vi "Github Demo Test VI.vi"() -> ()   [LabVIEW 2016]
uses:
  <vilib>/Utility/file.llb/Write Delimited Spreadsheet (DBL).vi
panel:
  in  "stop":bool
  out "x+y":dbl
  out "error out":errorcluster
  in  "file path":path
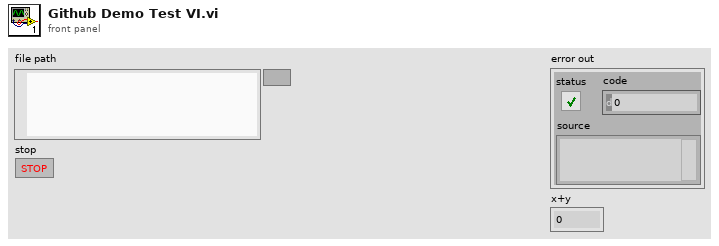
[diagram p1: front panel]
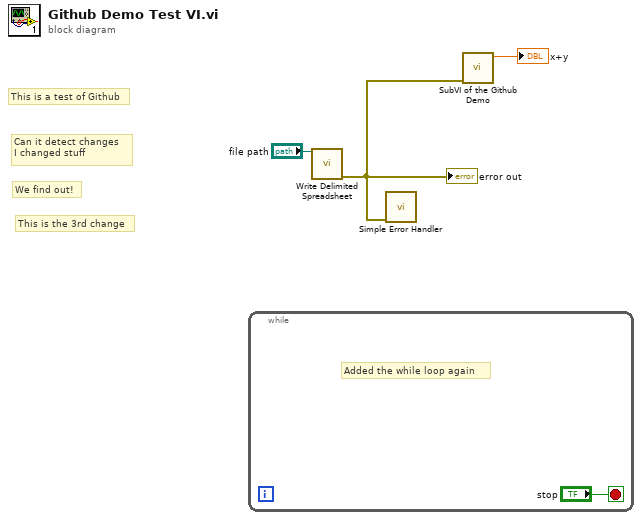
[diagram p0: block diagram]
diagram:
  # "This is the 3rd change"
  # "We find out!"
  # "Can it detect changes \nI changed stuff"
  # "This is a test of Github"
  n1 = while {
    stop <- "stop" stop-if-true
    # "Added the while loop again"
  }
  n2 = call-poly <vilib>:"Write Delimited Spreadsheet.vi"("file path (dialog if empty)"="file path") -> ("error out"=w2:errorcluster)  [unwired: 13 in, 1 out]
  "error out" <- w2
  n3 = call <vilib>:"Simple Error Handler.vi"("error in (no error)"=w2) -> ()  [unwired: 4 in, 5 out]
  n4 = call "SubVI of the Github Demo.vi"("error in (no error)"=w2) -> ("x+y"=→"x+y":dbl)  [unwired: 10 in]
